vi "Send.vi"(9 "Priority?":bool, 10 "Msg Strategy":refnum<class "Msg Strategy.lvclass">, 11 "Event Msg Type Strategy in":refnum<class "Event Msg Type Strategy.lvclass">) -> (0 "error out":errorcluster)   [LabVIEW 2021, in "jettl.lvlib" / "Msg Type Strategy.lvlib" / "Event Msg Type Strategy.lvclass"]
uses:
  Event Msg Type Strategy.lvclass
  Msg Strategy/Msg Strategy.lvclass
  <vilib>/event_ctls.llb/usereventprio.ctl
  Event Msg Type Strategy.lvclass/Event Msg Type Strategy.ctl
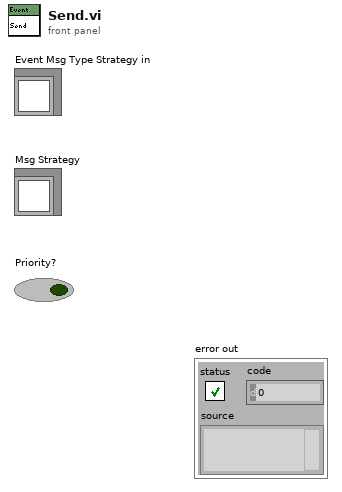
[diagram p1: front panel]
types:
  T1 = typedef "usereventprio.ctl" = enum32{"high priority", "normal priority"}
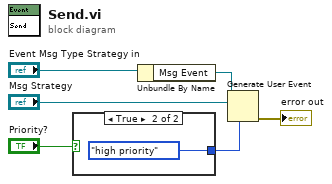
[diagram p0: block diagram]
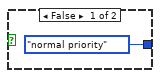
[diagram p2: hidden frame]
diagram:
  n1 = case shown="True" "Priority?" {
    tunnel: [usereventprio."normal priority" ("priority (normal)") usereventprio."high priority" ("priority (normal)")] -> w3
    frame False {
    }
    frame True {
    }
  }
  n2 = Unbundle By Name("Event Msg Type Strategy in") -> ("Msg Event"=w1:refnum<user-event>)
  n3 = Generate User Event(priority (normal)=w3, user event=w1, event data cluster="Msg Strategy") -> (error out=→"error out":errorcluster)  [unwired: 1 in, 1 out]
